vi "Shutdown.vi"(8 "error in (no error)":errorcluster, 11 "Stage_MadCityLab in":refnum<class "Stage_MadCityLab.lvclass">) -> (0 "error out":errorcluster, 3 "Stage_MadCityLab out":refnum<class "Stage_MadCityLab.lvclass">)   [LabVIEW 2020, in "Stage_MadCityLab.lvlib" / "Stage_MadCityLab.lvclass"]
uses:
  Stage_MadCityLab.lvclass
  Stage_MadCityLab.lvclass/Stage_MadCityLab.ctl
  Hardware Abstraction Layer/Component/Stage/Stage/Stage.lvclass
  Dependency/Madlib.dll
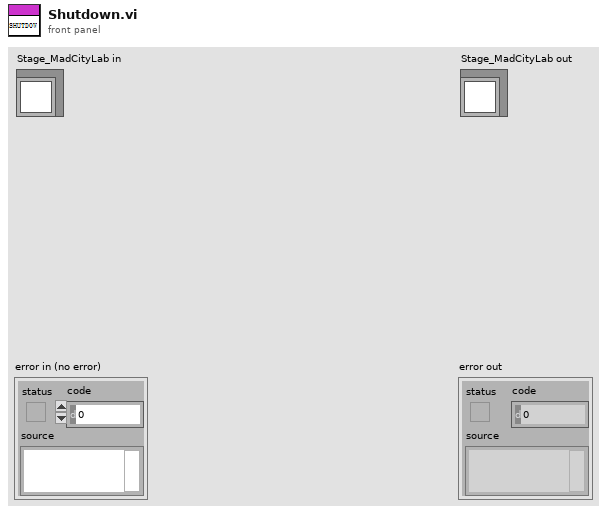
[diagram p1: front panel]
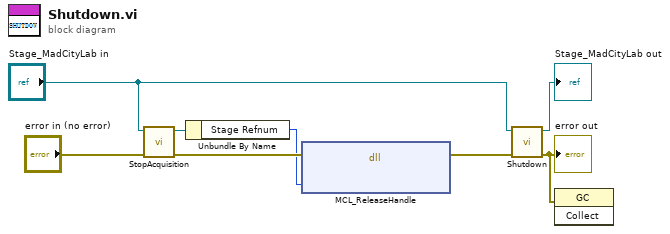
[diagram p0: block diagram]
diagram:
  n1 = call-dynamic "StopAcquisition.vi"("error in (no error)"="error in (no error)", "Device in"="Stage_MadCityLab in") -> ("error out"=w7:errorcluster, "Device out"=w3:refnum<class "Stage_MadCityLab.lvclass">)  [unwired: 8 in]
  n2 = Unbundle By Name(w3) -> ("Stage Refnum"=w4:i32)
  n3 = dll-call lib="E:/Development/DevHardSoftware/MicroscopyFramework/Model/Hardware Layer/Real Hardware/Stage_MadCityLab/Stage_MadCityLab/Dependency/Madlib.dll" fn="MCL_ReleaseHandle"(error in=w7, "handle"=w4) -> (error out=w6:errorcluster)  [unwired: 3 in, 2 out]
  n4 = call-parent "Shutdown.vi"("error in (no error)"=w6, "GRMActor in"="Stage_MadCityLab in") -> ("error out"=w5:errorcluster, "GRMActor out"=→"Stage_MadCityLab out":refnum<class "Stage_MadCityLab.lvclass">)  [unwired: 8 in]
  "error out" <- w5
  n5 = invoke class="GC" method="Collect"(error in=w5) -> ()  [unwired: 2 in, 3 out]
